vi "CFTS-Globals.vi"() -> ()   [LabVIEW 2020]
panel:
  in  "FP Controls":T1
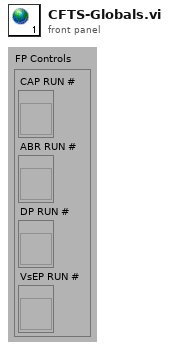
[diagram p1: front panel]
types:
  T1 = cluster{"CAP RUN #":refnum<vi>, "ABR RUN #":refnum<vi>, "DP RUN #":refnum<vi>, "VsEP RUN #":refnum<vi>}
diagram:
